vi "hw5_2_(1).vi"() -> ()   [LabVIEW 2014]
panel:
  in  "stop":bool
  out "Result":string
  in  "1":bool
  in  "+":bool
  in  "-":bool
  in  "/":bool
  in  "C":bool
  in  ".":bool
  in  "0":bool
  in  "backspace":bool
  in  "=":bool
  in  "*":bool
  in  "9":bool
  in  "8":bool
  in  "7":bool
  in  "6":bool
  in  "5":bool
  in  "4":bool
  in  "3":bool
  in  "2":bool
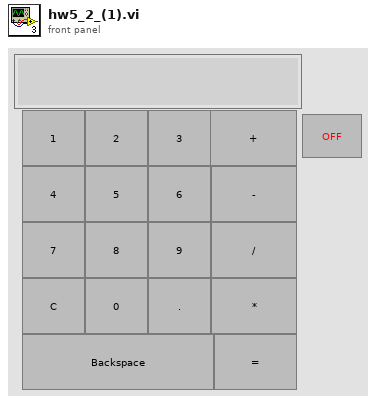
[diagram p1: front panel]
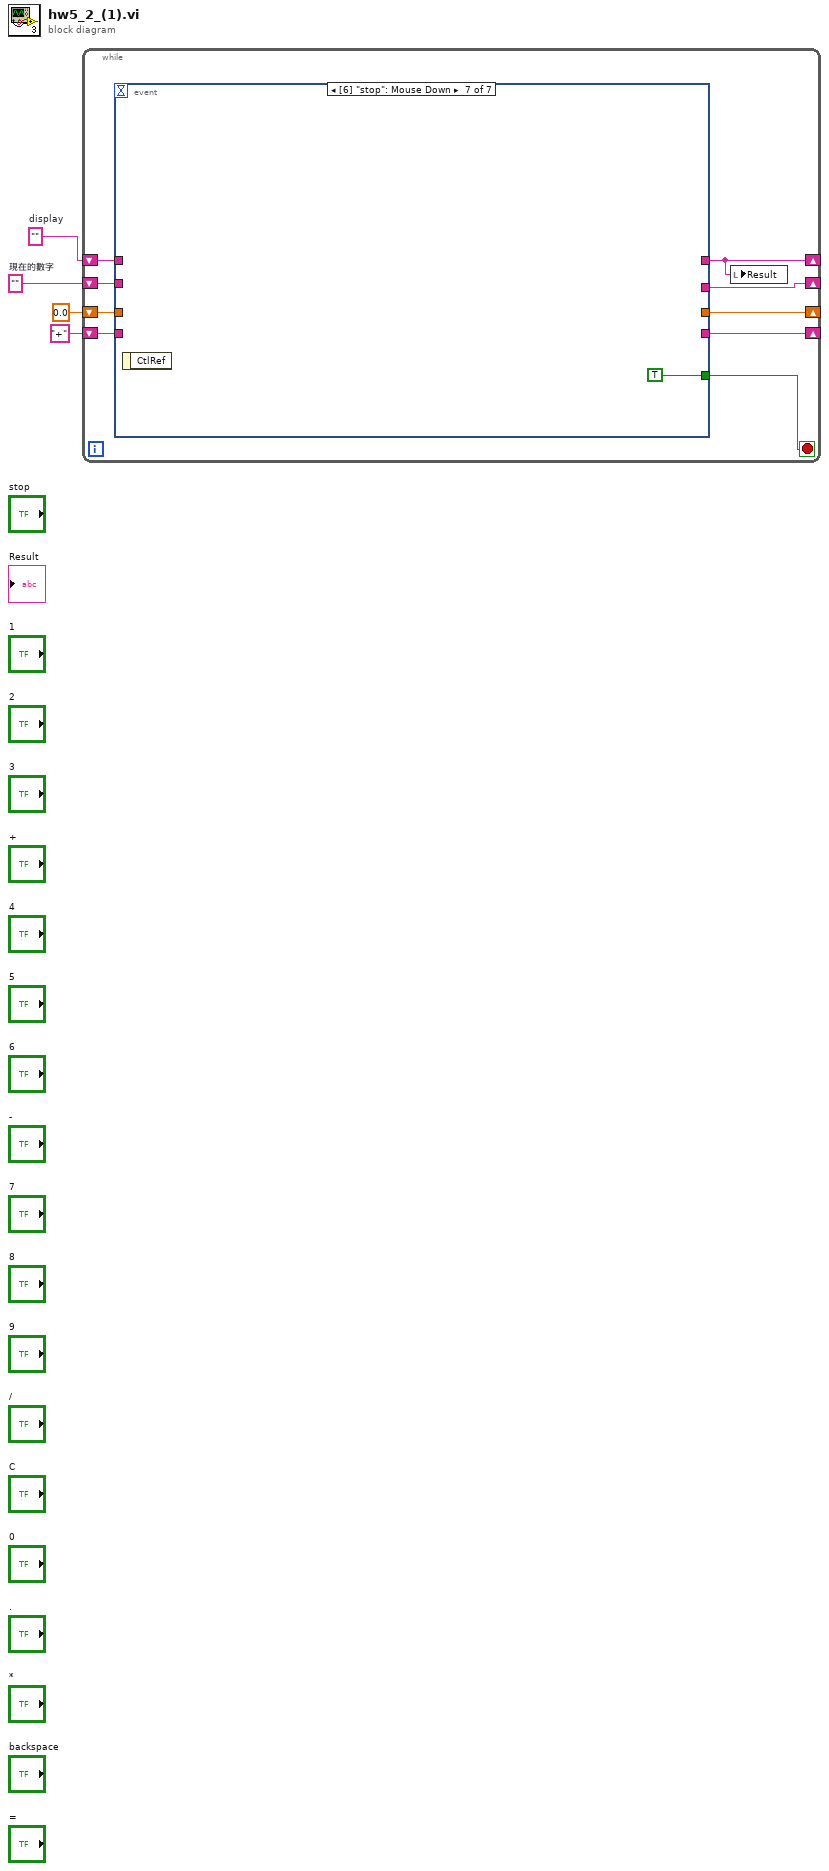
[diagram p0: block diagram]
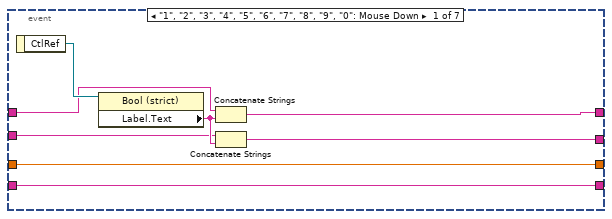
[diagram p2: hidden frame]
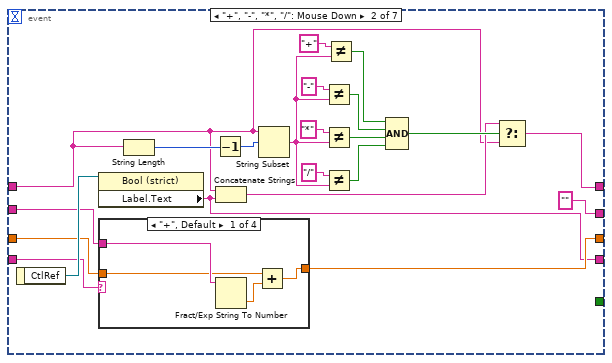
[diagram p3: hidden frame]
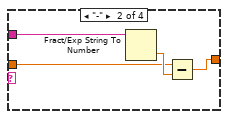
[diagram p4: hidden frame]
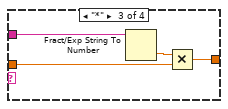
[diagram p5: hidden frame]
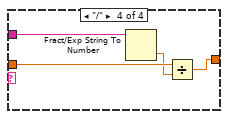
[diagram p6: hidden frame]
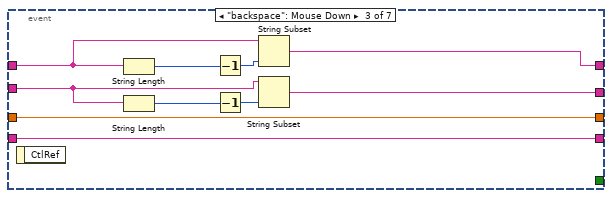
[diagram p7: hidden frame]
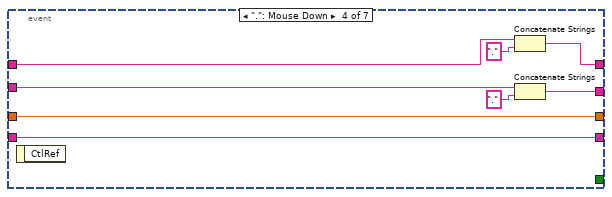
[diagram p8: hidden frame]
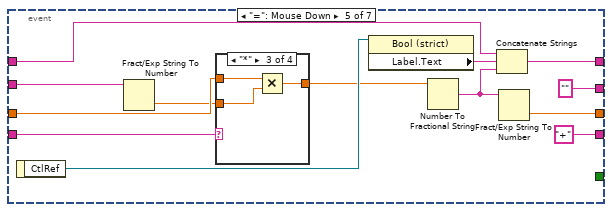
[diagram p9: hidden frame]
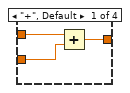
[diagram p10: hidden frame]
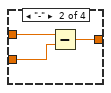
[diagram p11: hidden frame]
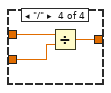
[diagram p12: hidden frame]
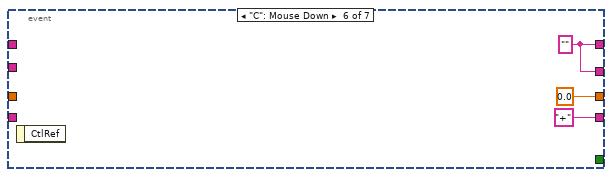
[diagram p13: hidden frame]
diagram:
  w3 = ""  # 現在的數字
  w4 = ""  # display
  n1 = while {
    shift-right: [w9] -> _
    shift-left: w4 -> [w13]
    shift-right: [w12] -> _
    shift-left: w3 -> [w11]
    shift-right: [w8] -> _
    shift-left: 0.0 -> [w10]
    shift-right: [w6] -> _
    shift-left: "+" -> [w7]
    stop <- w5 stop-if-true
    n2 = event shown="[6] \"stop\": Mouse Down" {
      selector: _ -> [_ _ _ _ _ _ _]
      dyn-events: _ -> [_ _ _ _ _ _ _]
      timeout: _ -> [_ _ _ _ _ _ _]
      tunnel: w13 -> [w20 w27 w66 w76 w88 _ _]
      tunnel: [w18 w29 w68 w73 w87 w105 _] -> w9
      tunnel: w10 -> [w19 w28 w64 w71 w81 _ _]
      tunnel: [w17 "" w61 w72 "" w105 _] -> w12
      tunnel: w11 -> [w15 w26 w60 w74 w86 _ _]
      tunnel: [w19 w24 w64 w71 w83 0.0 _] -> w8
      tunnel: w7 -> [w14 w23 w65 w70 w82 _ _]
      tunnel: [w14 w22 w65 w70 "+" "+" _] -> w6
      tunnel: [_ _ _ _ _ _ TRUE] -> w5
      event "1", "2", "3", "4", "5", "6", "7", "8", "9", "0": Mouse Down {
        n3 = event-data() -> ("CtlRef"=w21:refnum<vi>)  [unwired: 1 in]
        n4 = property class="Bool (strict)"(reference=w21) -> ("Label.Text"=w16:string)  [unwired: 1 in, 2 out]
        n5 = Concatenate Strings(w20, w16) -> (w18:string)
        n6 = Concatenate Strings(w15, w16) -> (w17:string)
      }
      event "+", "-", "*", "/": Mouse Down {
        n7 = event-data() -> ("CtlRef"=w43:refnum<vi>)  [unwired: 1 in]
        n8 = property class="Bool (strict)"(reference=w43) -> ("Label.Text"=w22:string)  [unwired: 1 in, 2 out]
        n9 = case shown="\"+\", Default" w23 {
          tunnel: w26 -> [w47 w51 w55 w59]
          tunnel: w28 -> [w44 w48 w53 w57]
          tunnel: [w46 w50 w54 w58] -> w24
          frame "+", Default {
            n10 = Fract/Exp String To Number(string=w47) -> (number=w45:dbl)  [unwired: 3 in, 1 out]
            n11 = Add(x=w44, y=w45) -> (x+y=w46:dbl)
          }
          frame "-" {
            n12 = Fract/Exp String To Number(string=w51) -> (number=w49:dbl)  [unwired: 3 in, 1 out]
            n13 = Subtract(x=w48, y=w49) -> (x-y=w50:dbl)
          }
          frame "*" {
            n14 = Fract/Exp String To Number(string=w55) -> (number=w52:dbl)  [unwired: 3 in, 1 out]
            n15 = Multiply(x=w52, y=w53) -> (x*y=w54:dbl)
          }
          frame "/" {
            n16 = Fract/Exp String To Number(string=w59) -> (number=w56:dbl)  [unwired: 3 in, 1 out]
            n17 = Divide(x=w57, y=w56) -> (x/y=w58:dbl)
          }
        }
        n18 = String Length(string=w27) -> (length=w42:i32)
        n19 = Decrement(x=w42) -> (x-1=w41:i32)
        n20 = Concatenate Strings(w27, w22) -> (w30:string)
        n21 = String Subset(string=w27, offset (0)=w41) -> (substring=w36:string)  [unwired: 1 in]
        n22 = Not Equal?(x="-", y=w36) -> (x != y?=w34:bool)
        n23 = Not Equal?(x="*", y=w36) -> (x != y?=w33:bool)
        n24 = Not Equal?(x="/", y=w36) -> (x != y?=w32:bool)
        n25 = Not Equal?(x="+", y=w36) -> (x != y?=w35:bool)
        n26 = Compound Arithmetic op=AND(w35, w34, w33, w32) -> (w31:bool)
        n27 = Select(t=w30, s=w31, f=w27) -> (s? t:f=w29:string)
      }
      event "backspace": Mouse Down {
        n28 = event-data() -> ()  [unwired: 1 in, 1 out]
        n29 = String Length(string=w66) -> (length=w69:i32)
        n30 = String Length(string=w60) -> (length=w63:i32)
        n31 = Decrement(x=w69) -> (x-1=w67:i32)
        n32 = Decrement(x=w63) -> (x-1=w62:i32)
        n33 = String Subset(string=w66, length (rest)=w67) -> (substring=w68:string)  [unwired: 1 in]
        n34 = String Subset(string=w60, length (rest)=w62) -> (substring=w61:string)  [unwired: 1 in]
      }
      event ".": Mouse Down {
        n35 = event-data() -> ()  [unwired: 1 in, 1 out]
        n36 = Concatenate Strings(w76, "." ("search string")) -> (w73:string)
        n37 = Concatenate Strings(w74, "." ("search string")) -> (w72:string)
      }
      event "=": Mouse Down {
        n38 = event-data() -> ("CtlRef"=w90:refnum<vi>)  [unwired: 1 in]
        n39 = Fract/Exp String To Number(string=w86) -> (number=w80:dbl)  [unwired: 3 in, 1 out]
        n40 = case shown="\"*\"" w82 {
          tunnel: w81 -> [w93 w96 w99 w102]
          tunnel: w80 -> [w92 w95 w98 w101]
          tunnel: [w91 w94 w97 w100] -> w79
          frame "+", Default {
            n41 = Add(x=w93, y=w92) -> (x+y=w91:dbl)
          }
          frame "-" {
            n42 = Subtract(x=w96, y=w95) -> (x-y=w94:dbl)
          }
          frame "*" {
            n43 = Multiply(x=w99, y=w98) -> (x*y=w97:dbl)
          }
          frame "/" {
            n44 = Divide(x=w102, y=w101) -> (x/y=w100:dbl)
          }
        }
        n45 = property class="Bool (strict)"(reference=w90) -> ("Label.Text"=w89:string)  [unwired: 1 in, 2 out]
        n46 = Number To Fractional String(number=w79) -> (F-format string=w84:string)  [unwired: 3 in]
        n47 = Concatenate Strings(w88, w89, w84) -> (w87:string)
        n48 = Fract/Exp String To Number(string=w84) -> (number=w83:dbl)  [unwired: 3 in, 1 out]
      }
      event "C": Mouse Down {
        w105 = ""
        n49 = event-data() -> ()  [unwired: 1 in, 1 out]
      }
      event "stop": Mouse Down {
        n50 = event-data() -> ()  [unwired: 1 in, 1 out]
      }
    }
    n51 = local write "Result"(w9) -> ()
  }
